vi "Flatten JSON Object to JSONpath Array.vi"(4 "Maximum Depth":i32=-1, 6 "Initial Path":string="$", 7 "Include $Paths to Objects":bool, 8 "error in (no error)":errorcluster, 10 "Offset":i32, 11 "JSON":string) -> (0 "error out":errorcluster, 1 "<JSON>":string[](array[string]) caption="<JSON>Items", 3 "$Paths":string[](array[string]))   [LabVIEW 2021, in "json.facade.lvlib"]
doc: "Takes a JSON Value and \"flattens\" the Object structure, producing out arrays of the $Paths to each item and the corresponding items. This works recursively on all subObjects (but not Arrays, which are treated as a single item).\n\nNote: to support names containing periods (.) in them, those names will be returned as a JSON string (quoted). \n\nFor example: the JSON {\"A\":{\"B1\":1,\"B2\":\"x\"},\"A2\":true,\"A.1\":{\"C\":123}} produces the arrays:\n$Paths (Items):\n$.A.B1 (1)\n$.A.B2 (\"x\")\n$.A2 (true)\n$.\"A.1\".C (123)\n\nIf \"Include $Paths to Objects\" is True, then the above list will incude a path to all Objects (including the root Object path \"$\"):\n$\n$.A\n$.A.B1\n$.A.B2\n$.A2\n$.\"A.1\"\n$.\"A.1\".C"
uses:
  json.facade.lvlib
  jsontext/JSONtext.lvlib
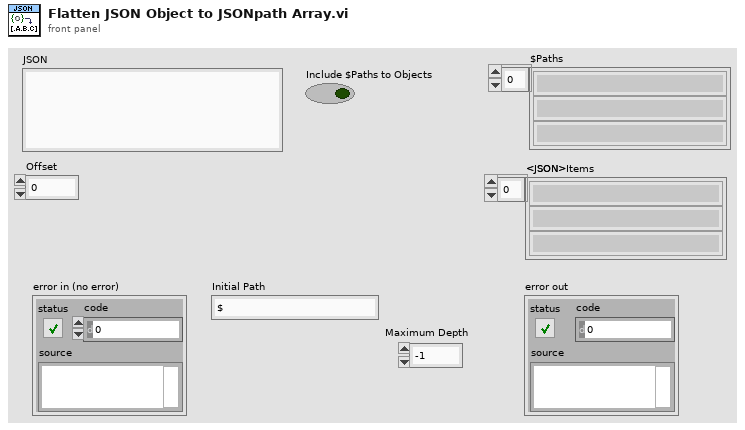
[diagram p1: front panel]
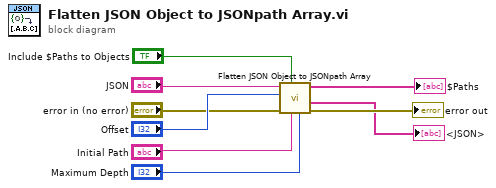
[diagram p0: block diagram]
diagram:
  n1 = call "Flatten JSON Object to JSONpath Array.vi"("Maximum Depth"="Maximum Depth", "Initial Path"="Initial Path", "Include $Paths to Objects"="Include $Paths to Objects", "error in (no error)"="error in (no error)", "Offset"="Offset", "JSON"="JSON") -> ("error out"=→"error out":errorcluster, "<JSON>"=→"<JSON>":string[], "$Paths"=→"$Paths":string[])  [unwired: 3 in]
